vi "XML Script - MathScriptNode.vi"(0 "name":string, 1 "typeindex":i32=-1, 2 "inputs":string[](array[string]), 3 "outputs":string[](array[string]), 4 "x":i32=-1, 5 "y":i32=-1, 6 "prefix (name)":string, 7 "functionName":string, 8 "IsODEUserFunction?":bool, 9 "functionPath":path, 11 "is dynamic?":bool, 12 "in":i32=-1, 13 "out":i32=-1) -> (14 "XML Script Command - MathScriptNode":string, 19 "name (wire source)":string)   [LabVIEW 2017]
uses:
  <vilib>/_script/XML Scripting/XML Script Attribute.ctl
  <vilib>/_script/XML Scripting/XML Script Tag.ctl
  <vilib>/_script/XML Scripting/XML Script - PathToXMLString.vi
panel:
  # "formula expression is passed\nthrough the array of variants"
  # "position"
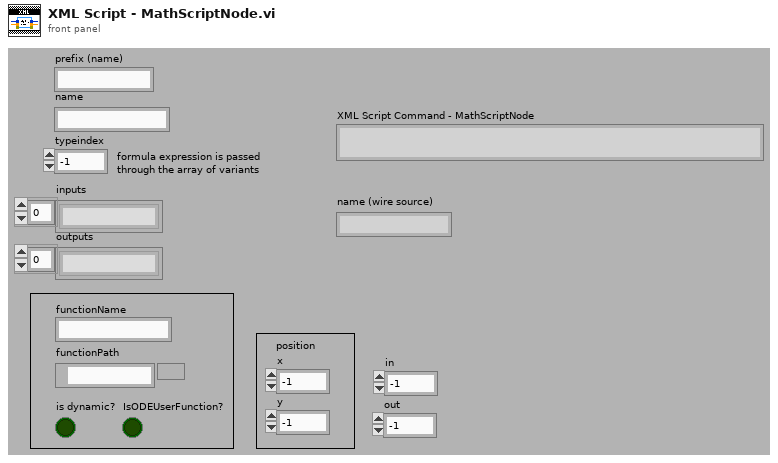
[diagram p1: front panel]
types:
  T1 = typedef "XML Script Attribute.ctl" = enum16{"name", "style", "path", "position", "in", "out", "width", "height", "index", "value", "default", "location", "offset", "typeindex", "size", "source", "destination", "indicator", "type", "controlname", "label", "conpaneidx", "mode", "description", "hasCondTerm", "linkIdentity", "caseselectortype", "concatInputs", "inName", "instantiationpath", "loopCondition", "IndexMode", "formulaInputs", "formulaOutputs", "msnFuncName", "msnIsDynamic", "msnIsODEUserFunction", "ignoreSearchDialog"}
  T2 = typedef "XML Script Tag.ctl" = enum16{"Script", "Function", "SubVI", "GrowableFunction", "Structure", "MultiframeStructure", "Frame", "Tunnel", "ShiftRegister", "Constant", "Control", "Terminal", "Wire", "StaticVIReference", "ControlTerminal", "CompoundArithmetic", "FlatSequence", "FlatSequenceFrame", "MathScriptCallByRef", "BuildArray", "GenericSubVI", "MathScriptNode"}
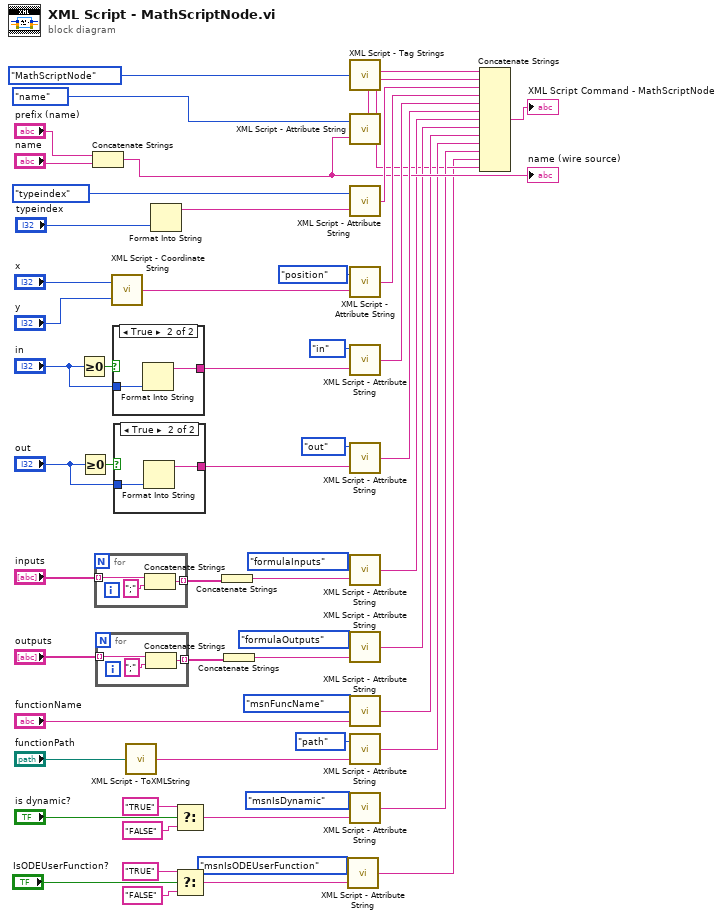
[diagram p0: block diagram]
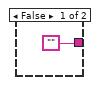
[diagram p2: hidden frame]
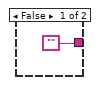
[diagram p3: hidden frame]
diagram:
  n1 = Greater Or Equal To 0?(x="in") -> (x >= 0?=w39:bool)
  n2 = Greater Or Equal To 0?(x="out") -> (x >= 0?=w43:bool)
  n3 = Concatenate Strings("prefix (name)", "name") -> (w35:string)
  "name (wire source)" <- w35
  n4 = for {
    tunnel: "inputs" -> [w60] mode=indexing
    tunnel: [w58] -> w31 mode=indexing
    n5 = Concatenate Strings(w60, ";" ("string")) -> (w58:string)
  }
  n6 = for {
    tunnel: "outputs" -> [w63] mode=indexing
    tunnel: [w61] -> w26 mode=indexing
    n7 = Concatenate Strings(w63, ";" ("string")) -> (w61:string)
  }
  n8 = call <vilib>:"XML Script - Coordinate String.vi"("y"="y", "x"="x") -> ("(x,y)"=w54:string)
  n9 = case shown="True" w39 {
    tunnel: "in" -> [_ w66]
    tunnel: ["" w65] -> w41
    frame False {
    }
    frame True {
      n10 = Format Into String(w66) -> (resulting string=w65:string)  [unwired: 3 in, 1 out]
    }
  }
  n11 = case shown="True" w43 {
    tunnel: "out" -> [_ w69]
    tunnel: ["" w68] -> w45
    frame False {
    }
    frame True {
      n12 = Format Into String(w69) -> (resulting string=w68:string)  [unwired: 3 in, 1 out]
    }
  }
  n13 = call-poly <vilib>:"XML Script - ToXMLString.vi"("Path"="functionPath") -> ("Valid XML String (out)"=w9:string)
  n14 = Format Into String("typeindex") -> (resulting string=w10:string)  [unwired: 3 in, 1 out]
  n15 = Select(t="TRUE", s="is dynamic?", f="FALSE") -> (s? t:f=w17:string)
  n16 = Select(t="TRUE", s="IsODEUserFunction?", f="FALSE") -> (s? t:f=w4:string)
  n17 = Concatenate Strings(w31) -> (w29:string)
  n18 = Concatenate Strings(w26) -> (w25:string)
  n19 = call <vilib>:"XML Script - Attribute String.vi"("Attribute String"=w4, "XML Script Attribute"=XML_Script_Attribute."msnIsODEUserFunction") -> ("XML Script - Attribute String"=w1:string)
  n20 = call <vilib>:"XML Script - Tag Strings.vi"("XML Script Tag"=XML_Script_Tag."MathScriptNode") -> ("XML String - Begin Tag"=w51:string, "XML String - End Tag"=w2:string)  [unwired: 2 in]
  n21 = call <vilib>:"XML Script - Attribute String.vi"("Attribute String"=w35, "XML Script Attribute"=XML_Script_Attribute."name") -> ("XML Script - Attribute String"=w49:string)
  n22 = call <vilib>:"XML Script - Attribute String.vi"("Attribute String"=w10, "XML Script Attribute"=XML_Script_Attribute."typeindex") -> ("XML Script - Attribute String"=w47:string)
  n23 = call <vilib>:"XML Script - Attribute String.vi"("Attribute String"=w54, "XML Script Attribute"=XML_Script_Attribute."position") -> ("XML Script - Attribute String"=w46:string)
  n24 = call <vilib>:"XML Script - Attribute String.vi"("Attribute String"=w41, "XML Script Attribute"=XML_Script_Attribute."in") -> ("XML Script - Attribute String"=w37:string)
  n25 = call <vilib>:"XML Script - Attribute String.vi"("Attribute String"=w45, "XML Script Attribute"=XML_Script_Attribute."out") -> ("XML Script - Attribute String"=w36:string)
  n26 = call <vilib>:"XML Script - Attribute String.vi"("Attribute String"=w29, "XML Script Attribute"=XML_Script_Attribute."formulaInputs") -> ("XML Script - Attribute String"=w28:string)
  n27 = call <vilib>:"XML Script - Attribute String.vi"("Attribute String"=w25, "XML Script Attribute"=XML_Script_Attribute."formulaOutputs") -> ("XML Script - Attribute String"=w23:string)
  n28 = call <vilib>:"XML Script - Attribute String.vi"("Attribute String"="functionName", "XML Script Attribute"=XML_Script_Attribute."msnFuncName") -> ("XML Script - Attribute String"=w20:string)
  n29 = call <vilib>:"XML Script - Attribute String.vi"("Attribute String"=w9, "XML Script Attribute"=XML_Script_Attribute."path") -> ("XML Script - Attribute String"=w19:string)
  n30 = call <vilib>:"XML Script - Attribute String.vi"("Attribute String"=w17, "XML Script Attribute"=XML_Script_Attribute."msnIsDynamic") -> ("XML Script - Attribute String"=w13:string)
  n31 = Concatenate Strings(w51, w49, w47, w46, w37, w36, w28, w23, w20, w19, w13, w1, w2) -> (→"XML Script Command - MathScriptNode":string)
